vi "Set Instrument.vi"(10 "HAL GOOP4.lvlib:Instrument":refnum<class "Instrument.lvclass">, 11 "Virt Instrument Base in":refnum<class "Virt Instr Local.lvclass">) -> (3 "Virt Instrument Base out":refnum<class "Virt Instr Local.lvclass">)   [LabVIEW 2023, in "HAL GOOP4.lvlib" / "Virt Instr Local.lvclass"]
uses:
  Virt Instr Local.lvclass
  Instrument/Instrument.lvclass
  Virt Instr Local.lvclass/Virt Instr Local.ctl
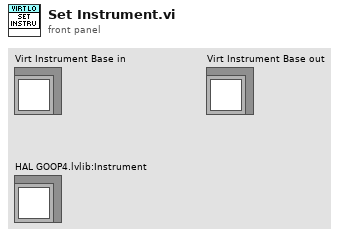
[diagram p1: front panel]
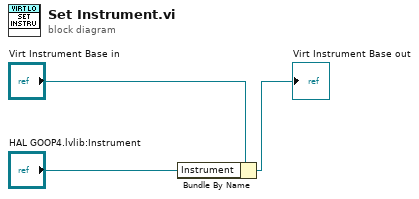
[diagram p0: block diagram]
diagram:
  n1 = Bundle By Name(cluster="Virt Instrument Base in", "Instrument"="HAL GOOP4.lvlib:Instrument") -> (→"Virt Instrument Base out":refnum<class "Virt Instr Local.lvclass">)
